vi "Init.vi"(8 "error in (no error)":errorcluster, 11 "Data in":refnum<class "Const_WFM.lvclass">) -> (0 "error out":errorcluster, 3 "Data out":refnum<class "Const_WFM.lvclass">)   [LabVIEW 2021, in "Const_WFM.lvclass"]
uses:
  Const_WFM.lvclass
  Const_WFM.lvclass/Const_WFM.ctl
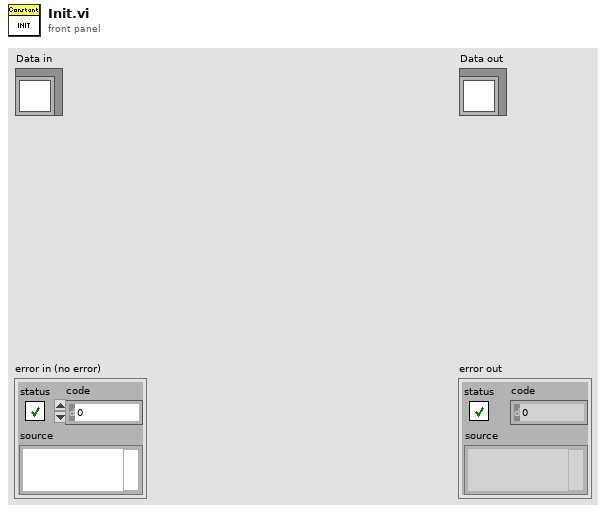
[diagram p1: front panel]
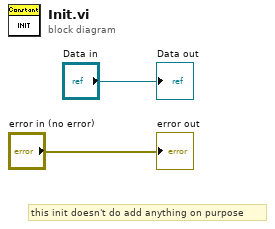
[diagram p0: block diagram]
diagram:
  # "this init doesn't do add anything on purpose"
  "error out" <- "error in (no error)"
  "Data out" <- "Data in"
